vi "node.vi"() -> ()   [LabVIEW 2020]
panel:
  in  "Array":bool[](array[boolean])
  in  "stop":bool
  out "Numeric 5":dbl
  out "Numeric 4":dbl
  out "Numeric 3":dbl
  out "Numeric 2":dbl
  out "Numeric":dbl
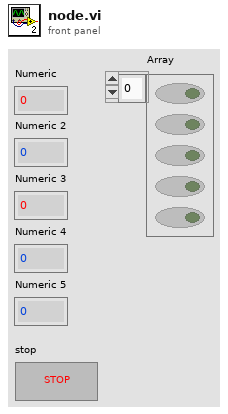
[diagram p1: front panel]
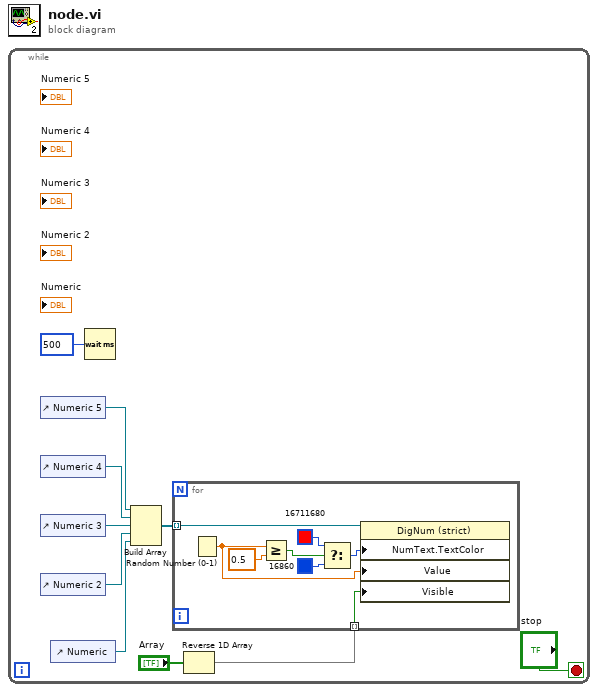
[diagram p0: block diagram]
diagram:
  n1 = while {
    stop <- "stop" stop-if-true
    n2 = control-ref of="Numeric 5"() -> (w8:refnum<vi>)
    n3 = control-ref of="Numeric 4"() -> (w7:refnum<vi>)
    n4 = control-ref of="Numeric 3"() -> (w6:refnum<vi>)
    n5 = control-ref of="Numeric 2"() -> (w5:refnum<vi>)
    n6 = control-ref of="Numeric"() -> (w4:refnum<vi>)
    n7 = Wait (ms)(milliseconds to wait=u32 500) -> ()  [unwired: 1 out]
    n8 = Build Array(w8, w7, w6, w5, w4) -> (w3:refnum<vi>[])
    n9 = Reverse 1D Array(array="Array") -> (reversed array=w1:bool[])
    n10 = for {
      tunnel: w3 -> [w13] mode=indexing
      tunnel: w1 -> [w11] mode=indexing
      n11 = Random Number (0-1)() -> (number: 0 to 1=w12:dbl)
      n12 = Greater Or Equal?(x=w12, y=0.5) -> (x >= y?=w17:bool)
      n13 = Select(t=u32 16711680 ("Numeric Text.Text Colors:Text Color"), s=w17, f=u32 16860 ("Numeric Text.Text Colors:Text Color")) -> (s? t:f=w16:u32)
      n14 = property class="DigNum (strict)"(reference=w13, "NumText.TextColor"=w16, "Value"=w12, "Visible"=w11) -> ()  [unwired: 1 in, 2 out]
    }
  }
